vi "RP-TRACKDataStructBuild.vi"(3 "CHANNELS PARAMETERS":T1[](array[typedef]) {"SPACING 2" min=0.0 max=100.0 step=0.5; "Points N° 2" min=0 max=100 step=1; "PROBE" min=0.0 max=100.0 step=0.5; "PUMP" min=0.0 max=100.0 step=0.5}, 4 "Track session name":string, 5 "SensWay track data path":path) -> (0 "TRACK REPOSITERY":path, 1 "Track File List":path[](array[path]), 2 "Track Repositery List":path[](array[path]))   [LabVIEW 2021]
uses:
  Channel parameters.ctl
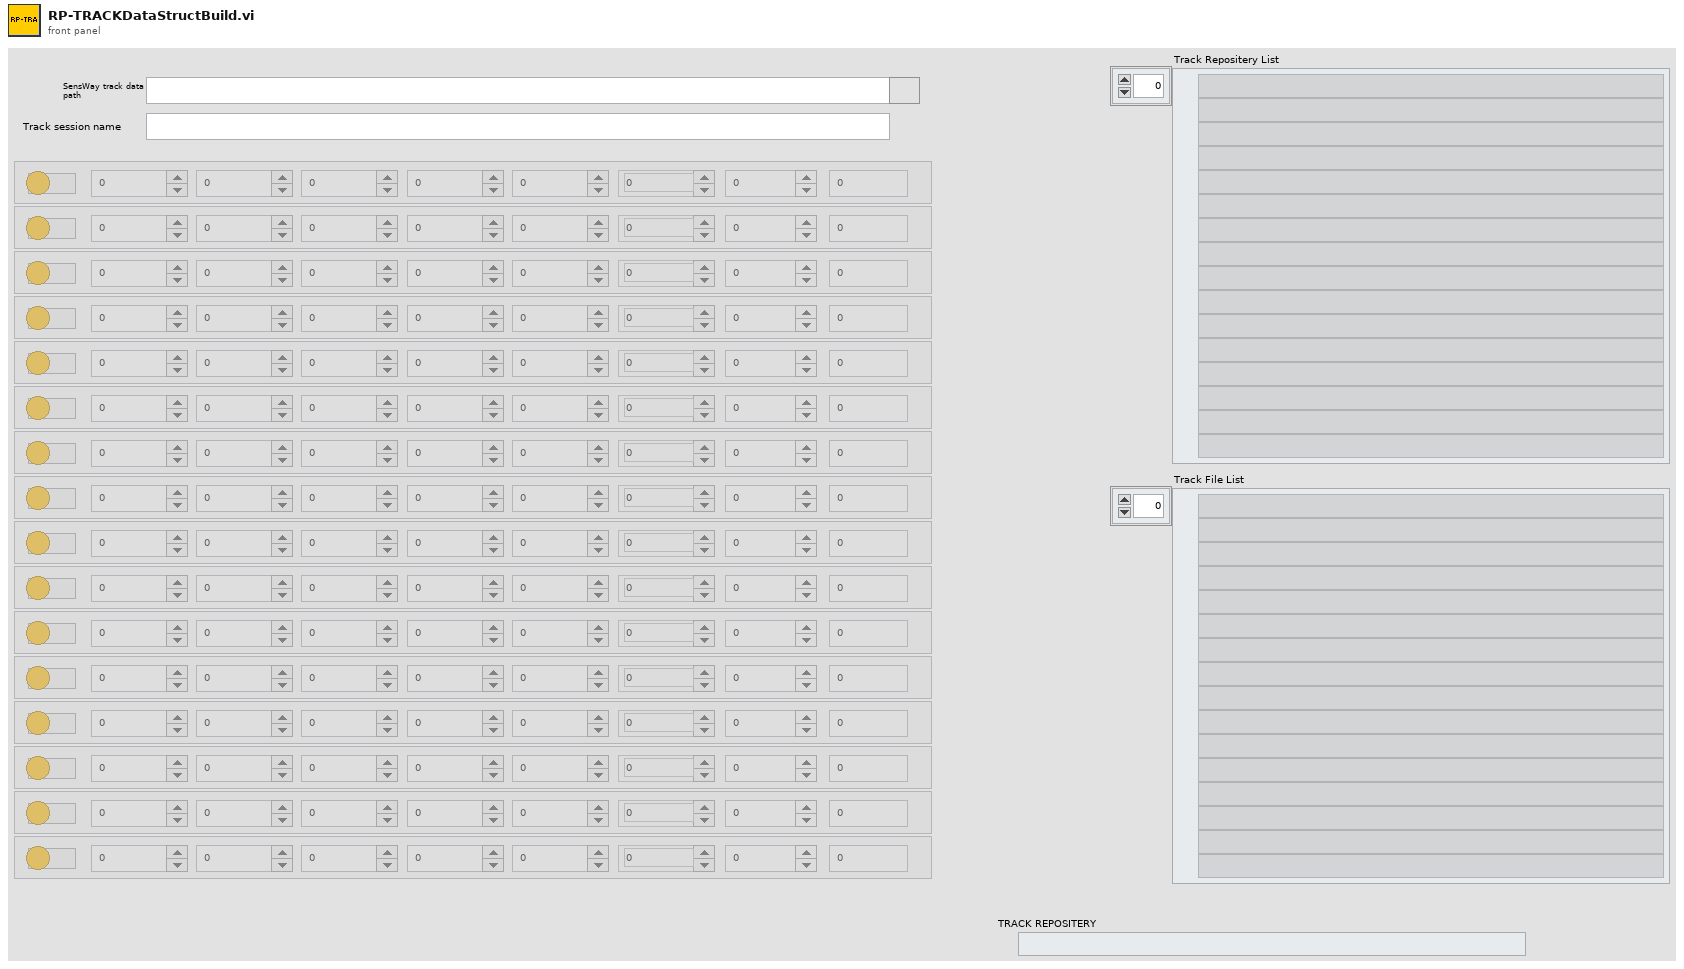
[diagram p1: front panel]
types:
  T1 = typedef "Channel parameters.ctl" = cluster{"START 2":dbl, "STOP 2":dbl, "CENTER 2":dbl, "SPAN 2":dbl, "CHANNEL TRACK ?":bool, "PUMP":dbl, "PROBE":dbl, "Points N° 2":i32, "SPACING 2":dbl}
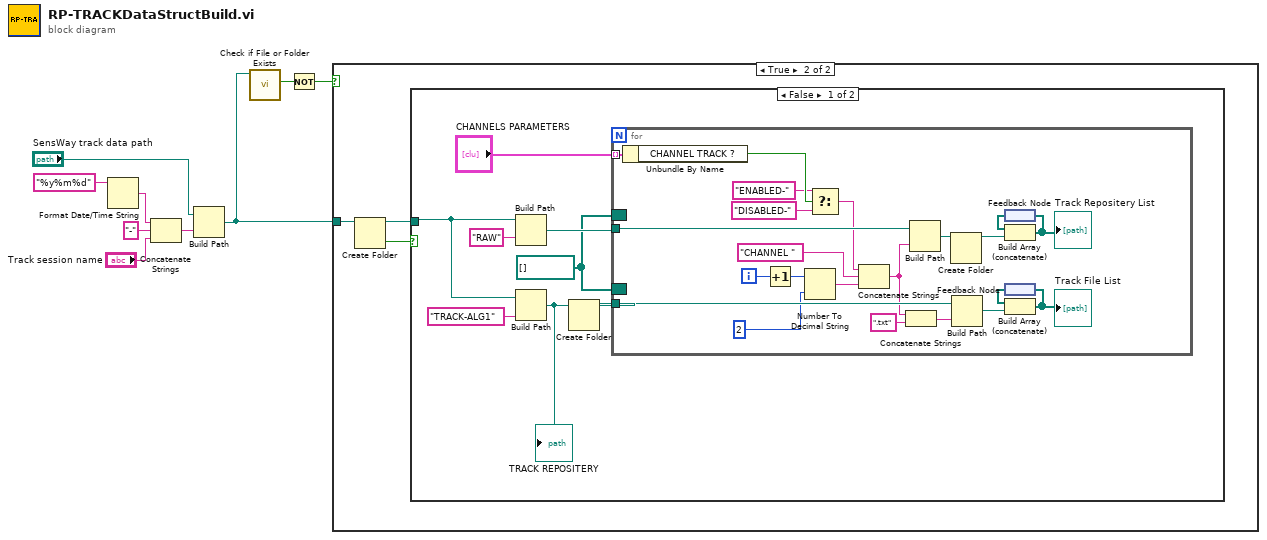
[diagram p0: block diagram]
diagram:
  n1 = Format Date/Time String(time format string (%c)="%y%m%d" ("chaîne de format de l'heure (%c)")) -> (date/time string=w7:string)  [unwired: 2 in]
  n2 = Concatenate Strings(w7, "-" ("Track session name 2"), "Track session name") -> (w9:string)
  n3 = Build Path(base path="SensWay track data path", name or relative path=w9) -> (appended path=w3:path)
  n4 = call <vilib>:"Check if File or Folder Exists.vi"("path"=w3) -> ("file or folder exists?"=w2:bool)  [unwired: 8 in, 2 out]
  n5 = Not(x=w2) -> (.not. x?=w1:bool)
  n6 = case shown="True" w1 {
    tunnel: w3 -> [_ w10]
    frame False {
    }
    frame True {
      n7 = Create Folder(path (use dialog)=w10) -> (created path=w12:path, cancelled=w11:bool)  [unwired: 2 in, 1 out]
      n8 = case shown="False" w11 {
        tunnel: w12 -> [w18 _]
        frame False {
          w15 = path[] []
          n9 = Build Path(base path=w18, name or relative path="RAW" ("Track session name 2")) -> (appended path=w16:path)
          n10 = Build Path(base path=w18, name or relative path="TRACK-ALG1" ("Track session name 2")) -> (appended path=w14:path)
          "TRACK REPOSITERY" <- w14
          n11 = Create Folder(path (use dialog)=w14) -> (created path=w13:path)  [unwired: 2 in, 2 out]
          n12 = for {
            tunnel: "CHANNELS PARAMETERS" -> [w42] mode=indexing
            tunnel: w16 -> [w41]
            tunnel: w13 -> [w40]
            border: w15 -> [_]
            border: w15 -> [_]
            i -> [w22]
            n13 = Unbundle By Name(w42) -> ("CHANNEL TRACK ?"=w26:bool)
            n14 = Increment(x=w22) -> (x+1=w21:i32)
            n15 = Number To Decimal String(number=w21, width (-)=i16 2) -> (decimal integer string=w39:string)
            n16 = Select(t="ENABLED-" ("string"), s=w26, f="DISABLED-" ("string")) -> (s? t:f=w23:string)
            n17 = Concatenate Strings(w23, "CHANNEL " ("string"), w39) -> (w37:string)
            n18 = Concatenate Strings(w37, ".txt" ("chaîne")) -> (w34:string)
            n19 = Build Path(base path=w41, name or relative path=w37) -> (appended path=w36:path)
            n20 = Create Folder(path (use dialog)=w36) -> (created path=w33:path)  [unwired: 2 in, 2 out]
            n21 = Build Path(base path=w40, name or relative path=w34) -> (appended path=w30:path)
            n22 = feedback #1() -> (w32:path[])
            n23 = Build Array (concatenate)(w32, w33) -> (w29:path[])
            "Track Repositery List" <- w29
            n24 = feedback-in #1(w29) -> ()
            n25 = feedback #2() -> (w31:path[])
            n26 = Build Array (concatenate)(w31, w30) -> (w28:path[])
            "Track File List" <- w28
            n27 = feedback-in #2(w28) -> ()
          }
        }
        frame True {
        }
      }
    }
  }
